vi "Set all f same.vi"(8 "error in (no error)":errorcluster, 10 "AO f":dbl, 11 "Instrument.Lockin":refnum<class "Instrument.Lockin.lvclass">) -> (0 "error out":errorcluster, 3 "Instrument.Lockin out":refnum<class "Instrument.Lockin.lvclass">)   [LabVIEW 2020, in "Instrument.Lockin.lvclass"]
uses:
  Instrument.Lockin.lvclass
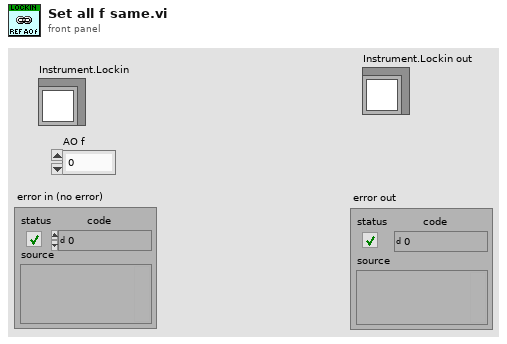
[diagram p1: front panel]
types:
  T1 = typedef "LockinDAQ.lvclass/AO-cluster.ctl" = cluster{"Ch":i32[], "Amp (V)":dbl[], "DC (V)":dbl[], "f (Hz)":dbl[], "Phase (°)":dbl[], "Function":T2[], "Sweep?":bool[]}
  T2 = typedef "LockinDAQ.lvclass/Function-enum.ctl" = enum16{"Sine", "Triangle", "Square", "Sawtooth"}
  T3 = typedef "LockinDAQ.lvclass/REF-cluster.ctl" = cluster{"Ch":i32[], " f (Hz)":dbl[], "Phase (°)":dbl[], "TC (s)":dbl[], "order":i32[]}
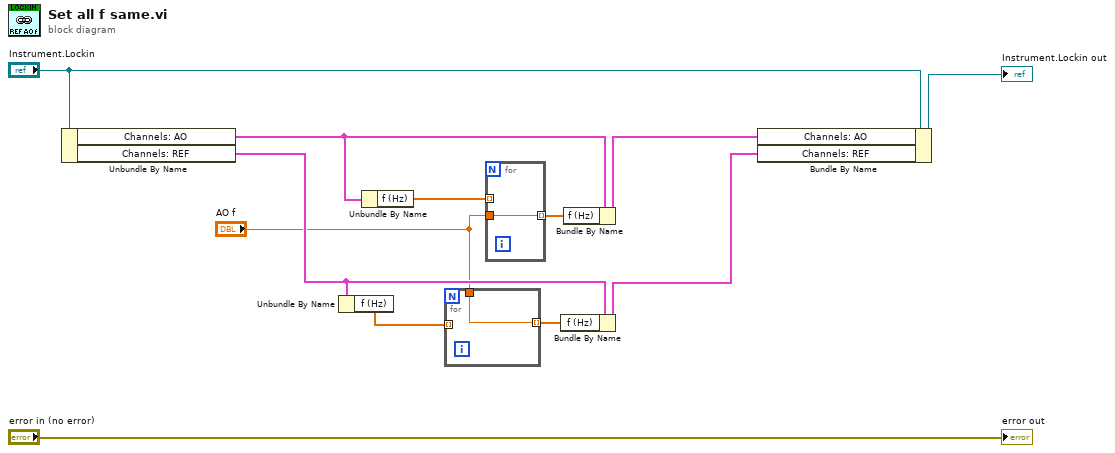
[diagram p0: block diagram]
diagram:
  n1 = Unbundle By Name("Instrument.Lockin") -> ("Channels: AO"=w2:T1, "Channels: REF"=w4:T3)
  n2 = Unbundle By Name(w4) -> ("f (Hz)"=w9:dbl[])
  n3 = Unbundle By Name(w2) -> ("f (Hz)"=w1:dbl[])
  n4 = for {
    tunnel: w9 -> [_] mode=indexing
    tunnel: [w13] -> w8 mode=indexing
    tunnel: "AO f" -> [w13]
  }
  n5 = for {
    tunnel: "AO f" -> [w14]
    tunnel: [w14] -> w7 mode=indexing
    tunnel: w1 -> [_] mode=indexing
  }
  n6 = Bundle By Name(cluster=w4, "f (Hz)"=w8) -> (w6:T3)
  n7 = Bundle By Name(cluster=w2, "f (Hz)"=w7) -> (w5:T1)
  n8 = Bundle By Name(cluster="Instrument.Lockin", "Channels: AO"=w5, "Channels: REF"=w6) -> (→"Instrument.Lockin out":refnum<class "Instrument.Lockin.lvclass">)
  "error out" <- "error in (no error)"
